vi "Append Subtopic.vi"(8 "error in (no error)":errorcluster, 10 "SubTopic In":refnum<class "Topic.lvclass">, 11 "Topic in":refnum<class "Topic.lvclass">) -> (0 "error out":errorcluster, 3 "Topic out":refnum<class "Topic.lvclass">)   [LabVIEW 2020, in "Topic.lvclass"]
uses:
  Topic.lvclass
  Topic.lvclass/Topic.ctl
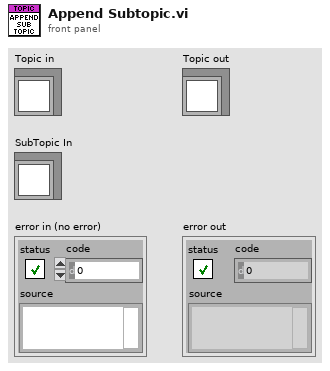
[diagram p1: front panel]
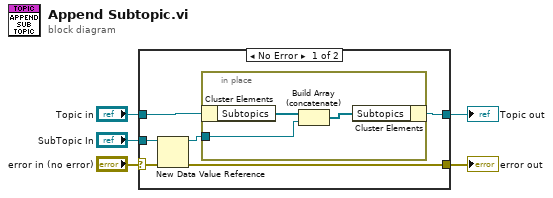
[diagram p0: block diagram]
diagram:
  n1 = case shown="No Error" "error in (no error)" {
    selector: "error in (no error)" -> [w7 w16]
    tunnel: [w6 w16] -> w4
    tunnel: [w10 w15] -> w2
    tunnel: "Topic in" -> [w11 w15]
    tunnel: "SubTopic In" -> [w8 _]
    frame No Error {
      n2 = New Data Value Reference(data value=w8, error in=w7) -> (data value reference=w9:refnum<data-value>, error out=w6:errorcluster)
      n3 = in-place {
        in-place-border: w9 -> [w13]
        n4 = in-place-cluster #1(w11) -> ("Subtopics"=w14:refnum<data-value>[])
        n5 = Build Array (concatenate)(w14, w13) -> (w12:refnum<data-value>[])
        n6 = in-place-cluster #1("Subtopics"=w12) -> (w10:refnum<class "Topic.lvclass">)
      }
    }
    frame Error {
    }
  }
  "error out" <- w4
  "Topic out" <- w2
